vi "Whether to Delete File.vi"(7 "Del Log file?":bool=TRUE, 8 "error in (no error)":errorcluster, 10 "Number of lines":i32, 11 "File path":path) -> (0 "error out":errorcluster)   [LabVIEW 2018]
uses:
  <vilib>/Utility/file.llb/Read Delimited Spreadsheet (string).vi
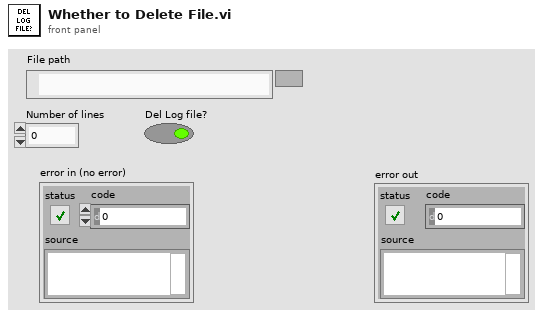
[diagram p1: front panel]
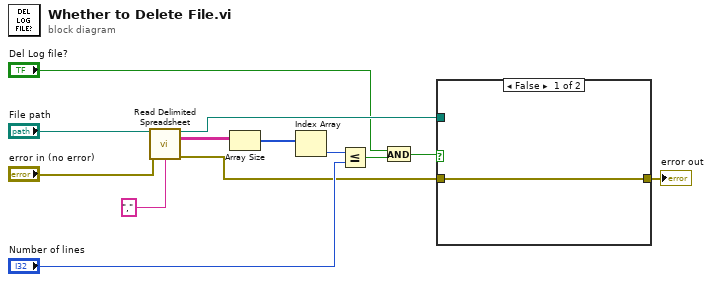
[diagram p0: block diagram]
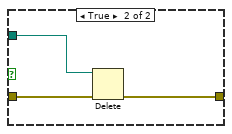
[diagram p2: hidden frame]
diagram:
  n1 = call-poly <vilib>:"Read Delimited Spreadsheet.vi"("file path (dialog if empty)"="File path", "error in (no error)"="error in (no error)", "delimiter (\\t)"="," ("delimiter (\\t)")) -> ("new file path (Not A Path if cancelled)"=w5:path, "all rows"=w11:string[][], "error out"=w6:errorcluster)  [unwired: 7 in, 3 out]
  n2 = Array Size(array=w11) -> (size(s)=w10:i32[])
  n3 = Index Array(array=w10) -> (element=w9:i32)  [unwired: 1 in]
  n4 = Less Or Equal?(x=w9, y="Number of lines") -> (x <= y?=w3:bool)
  n5 = And(x="Del Log file?", y=w3) -> (x .and. y?=w1:bool)
  n6 = case shown="False" w1 {
    tunnel: w6 -> [w14 w17]
    tunnel: w5 -> [_ w16]
    tunnel: [w14 w15] -> w4
    frame False {
    }
    frame True {
      n7 = Delete(path (use dialog)=w16, error in=w17) -> (error out=w15:errorcluster)  [unwired: 3 in, 2 out]
    }
  }
  "error out" <- w4
